vi "Destroy Sync Refnums.vi"(8 "error in":errorcluster) -> (0 "error out":errorcluster)   [LabVIEW 2026, in "Servo Motor Emulator.lvlib"]
doc: "Destroy the sync refnums used to synchronize event generation and event registration between the module and its caller(s).\n_____\nBased on DQMH Dev Tools: Project Template 7.1.2.1547."
uses:
  Servo Motor Emulator.lvlib
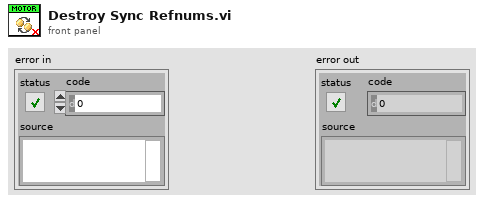
[diagram p1: front panel]
types:
  T1 = typedef "Rendezvous RefNum" = refnum<k1>
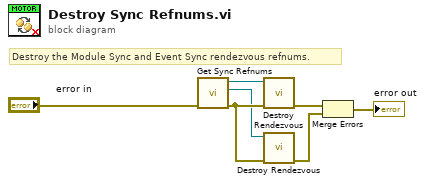
[diagram p0: block diagram]
diagram:
  # "Destroy the Module Sync and Event Sync rendezvous refnums."
  n1 = call "Get Sync Refnums.vi"("error in"="error in") -> ("error out"=w7:errorcluster, "Event Sync"=w3:T1, "Module Sync"=w5:T1)  [unwired: 8 in]
  n2 = call <vilib>:"Destroy Rendezvous.vi"("error in (no error)"=w7, "rendezvous"=w5) -> ("error out"=w4:errorcluster)  [unwired: 4 in, 1 out]
  n3 = call <vilib>:"Destroy Rendezvous.vi"("error in (no error)"=w7, "rendezvous"=w3) -> ("error out"=w1:errorcluster)  [unwired: 4 in, 1 out]
  n4 = Merge Errors(w4, w1) -> (→"error out":errorcluster)
